vi "add_sub_vi.vi"(8 "error in (no error)":errorcluster, 9 "SubVI":refnum<class "HierarchyNode.lvclass">, 10 "VI":refnum<class "HierarchyNode.lvclass">, 11 "VIHierarchyGraph in":refnum<class "HierarchyGraph.lvclass">) -> (0 "error out":errorcluster, 3 "VIHierarchyGraph out":refnum<class "HierarchyGraph.lvclass">)   [LabVIEW 2020, in "vi-hierarchy.lvlib" / "HierarchyGraph.lvclass"]
uses:
  HierarchyGraph.lvclass
  Y:/FlowRails/lv-graph/source/api/DiGraph/DiGraph.lvclass
  VINode/HierarchyNode.lvclass
  Y:/FlowRails/lv-graph/source/api/Node/Node.lvclass
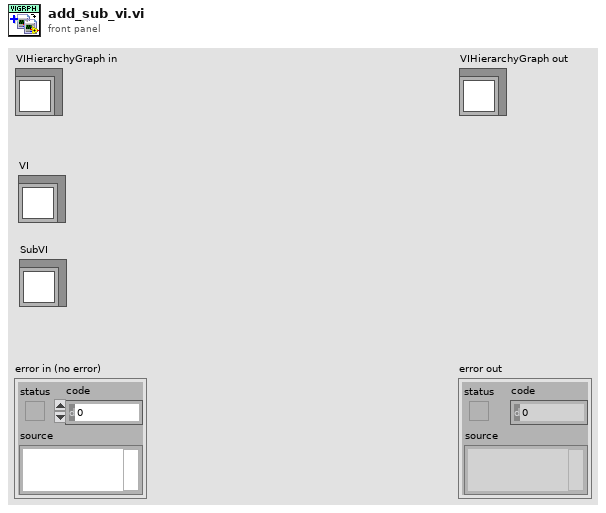
[diagram p1: front panel]
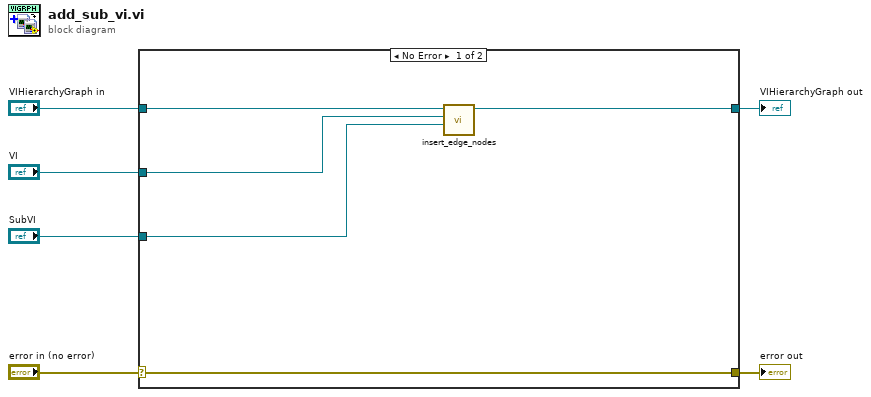
[diagram p0: block diagram]
diagram:
  n1 = case shown="No Error" "error in (no error)" {
    selector: "error in (no error)" -> [w7 w13]
    tunnel: [w7 w13] -> w5
    tunnel: [w11 w12] -> w3
    tunnel: "VIHierarchyGraph in" -> [w10 w12]
    tunnel: "VI" -> [w9 _]
    tunnel: "SubVI" -> [w8 _]
    frame No Error {
      n2 = call "insert_edge_nodes.vi"("destination-node"=w8, "source-node"=w9, "digraph"=w10) -> ("digraph out"=w11:refnum<class "HierarchyGraph.lvclass">)  [unwired: 6 in, 2 out]
    }
    frame Error {
    }
  }
  "error out" <- w5
  "VIHierarchyGraph out" <- w3
